vi "Drive_1.vi"(6 "Rotation":dbl, 7 "Gyro Angle":dbl, 8 "error in (no error)":errorcluster, 9 "Y":dbl, 10 "X":dbl, 11 "RobotDriveDevRef 2":T1={"DevStatus"={"status"=FALSE, "code"=0, "source"=""}, "Motors[]"=[], "Square Inputs"=FALSE, "Max Output"=1.0}) -> (0 "error out":errorcluster, 2 "Motor Values":dbl[](array[numeric]), 3 "RobotDriveDevRef":T1={"DevStatus"={"status"=FALSE, "code"=0, "source"=""}, "Motors[]"=[], "Square Inputs"=FALSE, "Max Output"=1.0})   [LabVIEW 2016]
uses:
  <vilib>/Rock Robotics/WPI/RobotDrive/WPI_RobotDriveDevRef.ctl
  <vilib>/Rock Robotics/WPI/MotorControl/WPI_MotorControlDeviceRef.ctl
  <vilib>/Rock Robotics/WPI/MotorControl/WPI_MotorControlType.ctl
  <vilib>/Rock Robotics/SystemInterfaces/DIO/FPGA_DIOPWMChannel.ctl
  <vilib>/Rock Robotics/WPI/PWM/WPI_PWMDeadband.ctl
  <vilib>/Rock Robotics/SystemInterfaces/NetworkCommunication/NetComm_UsageReport_ResourceType.ctl
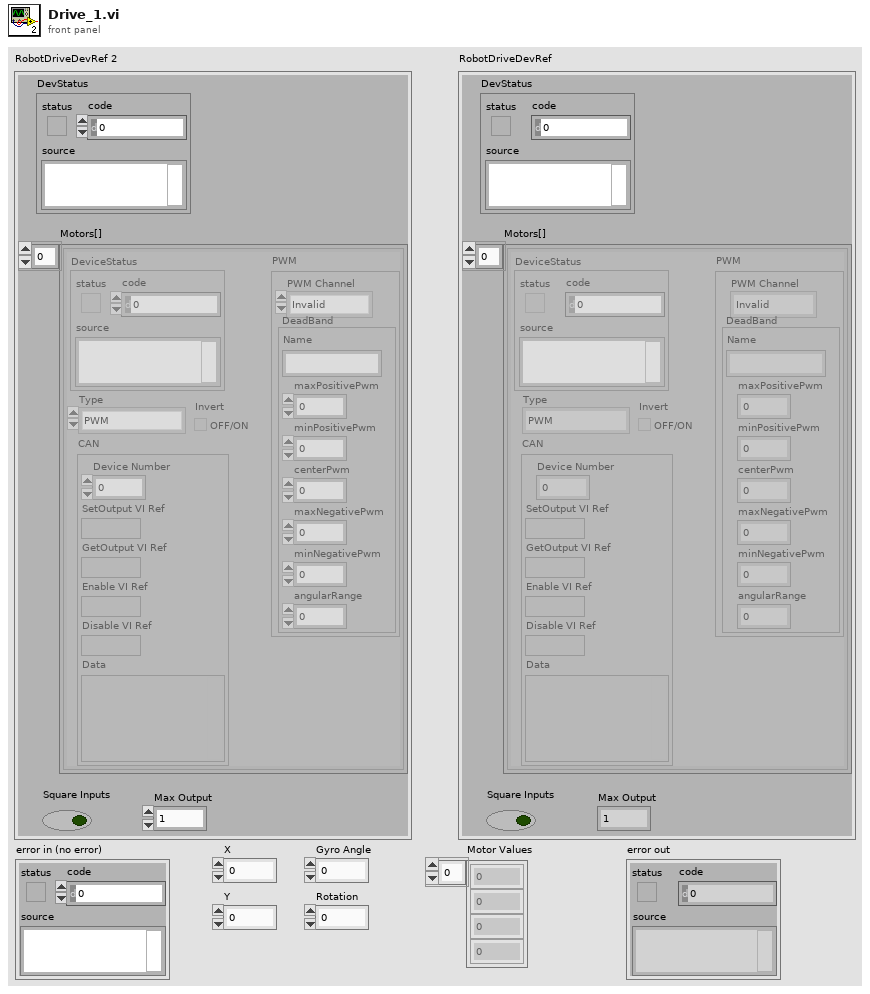
[diagram p1: front panel]
types:
  T1 = typedef "WPI_RobotDriveDevRef.ctl" = cluster{"DevStatus":errorcluster, "Motors[]":T2[], "Square Inputs":bool, "Max Output":dbl}
  T2 = typedef "WPI_MotorControlDeviceRef.ctl" = cluster{"DeviceStatus":errorcluster, "Type":T3, "PWM":cluster{"PWM Channel":T4, "DeadBand":T5}, "CAN":cluster{"Device Number":u8, "SetOutput VI Ref":variant, "GetOutput VI Ref":variant, "Enable VI Ref":variant, "Disable VI Ref":variant, "Data":variant}, "Invert":bool}
  T3 = typedef "WPI_MotorControlType.ctl" = enum16{"PWM", "CAN"}
  T4 = typedef "FPGA_DIOPWMChannel.ctl" = enum8{"PWM 0", "PWM 1", "PWM 2", "PWM 3", "PWM 4", "PWM 5", "PWM 6", "PWM 7", "PWM 8", "PWM 9", "PWM MXP 0", "PWM MXP 1", "PWM MXP 2", "PWM MXP 3", "PWM MXP 4", "PWM MXP 5", "PWM MXP 6", "PWM MXP 7", "PWM MXP 8", "PWM MXP 9", "Invalid"}
  T5 = typedef "WPI_PWMDeadband.ctl" = cluster{"Name":string, "maxPositivePwm":i32, "minPositivePwm":i32, "centerPwm":i32, "maxNegativePwm":i32, "minNegativePwm":i32, "angularRange":u16}
  T6 = typedef "NetComm_UsageReport_ResourceType.ctl" = enum8{"Controller", "Module", "Language", "CANPlugin", "Accelerometer", "ADXL345", "AnalogChannel", "AnalogTrigger", "AnalogTriggerOutput", "CANJaguar", "Compressor", "Counter", "Dashboard", "DigitalInput", "DigitalOutput", "DriverStationCIO", "DriverStationEIO", "DriverStationLCD", "Encoder", "GearTooth", "Gyro", "I2C", "Framework", "Jaguar", "Joystick", "Kinect", "KinectStick", "PIDController", "Preferences", "PWM", "Relay", "RobotDrive", "SerialPort", "Servo", "Solenoid", "SPI", "Task", "Ultrasonic", "Victor", "Button", "Command", "AxisCamera", "PCVideoServer", "SmartDashboard", "Talon", "HiTechnicColorSensor", "HiTechnicAccel", "HiTechnicCompass", "SRF08", "AnalogOutput", "Victor SP", "Talon SRX", "CAN Talon SRX", "ADXL362 Accel", "ADXRS450 Gyro", "Rev SPARK", "Mindsensors SD540", "Digital Filter", "ADIS16448", "PDP", "PCM", "PigeonIMU"}
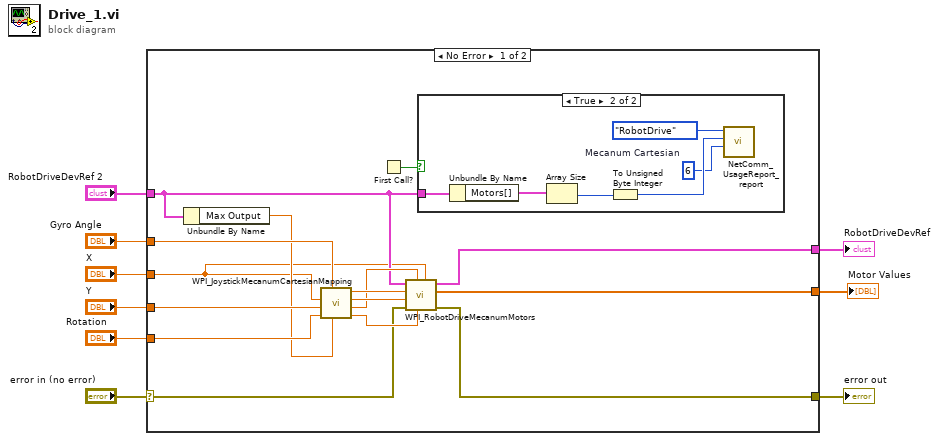
[diagram p0: block diagram]
diagram:
  n1 = case shown="No Error" "error in (no error)" {
    selector: "error in (no error)" -> [w13 w32]
    tunnel: "Y" -> [w22 _]
    tunnel: "X" -> [w10 _]
    tunnel: "RobotDriveDevRef 2" -> [w12 w31]
    tunnel: [w14 w31] -> w5
    tunnel: [w15 w32] -> w6
    tunnel: "Rotation" -> [w23 _]
    tunnel: "Gyro Angle" -> [w21 _]
    tunnel: [w16 _] -> w9
    frame No Error {
      n2 = Unbundle By Name(w12) -> ("Max Output"=w11:dbl)
      n3 = call <vilib>:"WPI_JoystickMecanumCartesianMapping.vi"("Max Output"=w11, "Gyro Angle"=w21, "Rotation"=w23, "Y"=w22, "X"=w10) -> ("Rear Right"=w20:dbl, "Rear Left"=w17:dbl, "Front Right"=w19:dbl, "Front Left"=w18:dbl)  [unwired: 3 in]
      n4 = First Call?() -> (First Call?: T/F=w24:bool)
      n5 = call <vilib>:"WPI_RobotDriveMecanumMotors.vi"("x"=w10, "Rear Right"=w20, "Rear Left"=w17, "error in"=w13, "Front Right"=w19, "Front Left"=w18, "RobotDriveDevRef in"=w12) -> ("error out"=w15:errorcluster, "Motor Values"=w16:dbl[], "RobotDriveDevRef out"=w14:T1)  [unwired: 2 in]
      n6 = case shown="True" w24 {
        tunnel: w12 -> [_ w25]
        frame False {
        }
        frame True {
          w28 = u8 6  # Mecanum Cartesian
          n7 = Unbundle By Name(w25) -> ("Motors[]"=w27:T2[])
          n8 = Array Size(array=w27) -> (size(s)=w26:i32)
          n9 = To Unsigned Byte Integer(number=w26) -> (unsigned 8bit integer=w29:u8)
          n10 = call <vilib>:"NetComm_UsageReport_report.vi"("Context"=w28, "Instance Number"=w29, "Resource Type"=NetComm_UsageReport_ResourceType."RobotDrive") -> ()  [unwired: 9 in]
        }
      }
    }
    frame Error {
    }
  }
  "error out" <- w6
  "RobotDriveDevRef" <- w5
  "Motor Values" <- w9
